vi "resetControl.vi"(0 "Interface in":T1, 11 "error in":errorcluster) -> (4 "Interface out":T1, 15 "error out":errorcluster)   [LabVIEW 2017, in "AFE_interface.lvlib"]
uses:
  AFE_interface.lvlib
  InterfaceRef.ctl
  <instrlib>/_niInstr/Instruction Framework/v1/Host/Instruction Target/niInstr Instruction Target v1 Host.lvclass
  <instrlib>/_niInstr/Instruction Framework/v1/Host/Instruction Framework Context/niInstr Instruction Framework Context v1 Host.lvclass
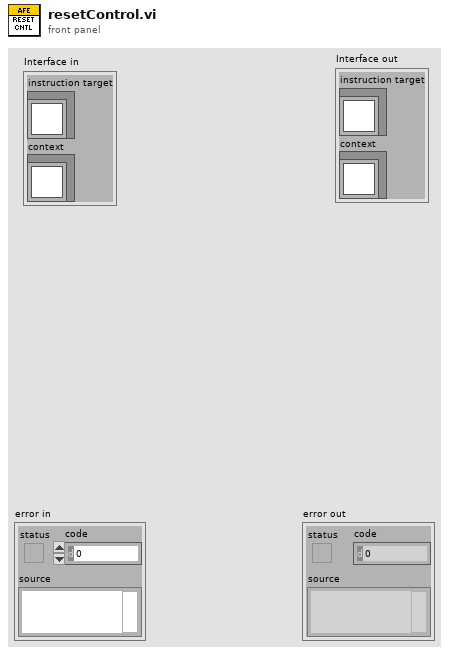
[diagram p1: front panel]
types:
  T1 = typedef "AFE_interface.lvlib/InterfaceRef.ctl" = cluster{"instruction target":refnum<class "niInstr Instruction Target v1 Host.lvclass">, "context":refnum<class "niInstr Instruction Framework Context v1 Host.lvclass">}
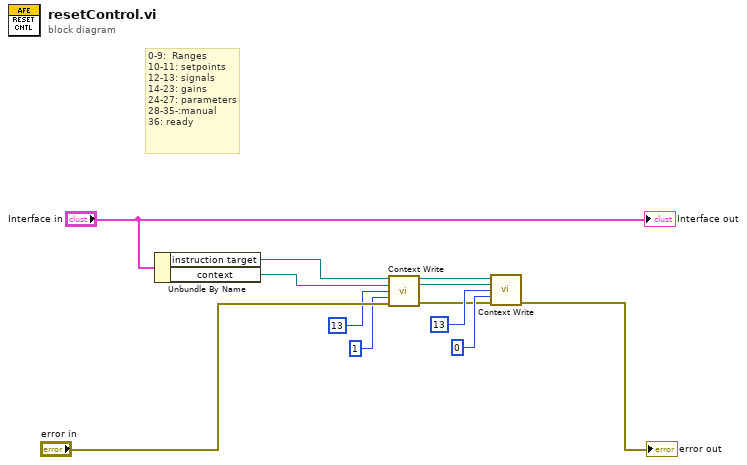
[diagram p0: block diagram]
diagram:
  # "0-9:  Ranges\n10-11: setpoints\n12-13: signals\n14-23: gains\n24-27: parameters\n28-35-:manual\n36: ready"
  n1 = Unbundle By Name("Interface in") -> ("instruction target"=w11:refnum<class "niInstr Instruction Target v1 Host.lvclass">, "context"=w10:refnum<class "niInstr Instruction Framework Context v1 Host.lvclass">)
  n2 = call <instrlib>:"Context Write.vi"("instruction target in"=w11, "context in"=w10, "address"=13 ("y"), "data"=u64 1, "error in"="error in") -> ("instruction target out"=w4:refnum<class "niInstr Instruction Target v1 Host.lvclass">, "context out"=w1:refnum<class "niInstr Instruction Framework Context v1 Host.lvclass">, "error out"=w3:errorcluster)  [unwired: 8 in]
  n3 = call <instrlib>:"Context Write.vi"("instruction target in"=w4, "context in"=w1, "address"=13 ("y"), "data"=u64 0, "error in"=w3) -> ("error out"=→"error out":errorcluster)  [unwired: 8 in, 2 out]
  "Interface out" <- "Interface in"
